vi "cleanWaypoints.vi"(10 "Waypoint Queue":refnum<queue>, 11 "Old Waypoints":refnum<class "Waypoint.lvclass">[](array[class])) -> (2 "Done?":bool, 3 "Old Waypoints (updated)":refnum<class "Waypoint.lvclass">[](array[class]))   [LabVIEW 2013]
doc: "When the next waypoints has been marked done, remove it from the queue and add it to the waypoint history array"
uses:
  Logic/Classes/Waypoint/Waypoint.lvclass
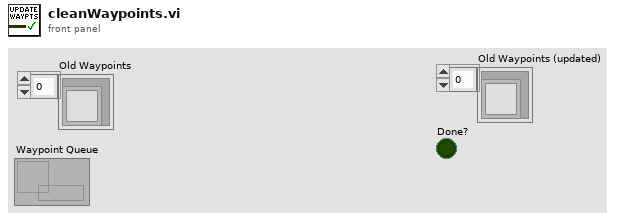
[diagram p1: front panel]
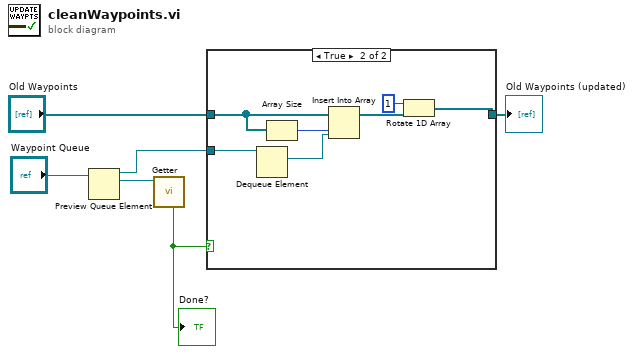
[diagram p0: block diagram]
diagram:
  n1 = Preview Queue Element(queue="Waypoint Queue") -> (queue out=w3:refnum<queue>, element=w5:refnum<class "Waypoint.lvclass">)  [unwired: 2 in, 2 out]
  n2 = call "Getter.vi"("Waypoint In"=w5) -> ("Done?"=w4:bool)  [unwired: 6 in, 4 out]
  "Done?" <- w4
  n3 = case shown="True" w4 {
    tunnel: w3 -> [_ w14]
    tunnel: "Old Waypoints" -> [w7 w12]
    tunnel: [w7 w8] -> w1
    frame False {
    }
    frame True {
      n4 = Dequeue Element(queue=w14) -> (element=w13:refnum<class "Waypoint.lvclass">)  [unwired: 2 in, 3 out]
      n5 = Array Size(array=w12) -> (size(s)=w11:i32)
      n6 = Insert Into Array(array=w12, index=w11, new element=w13) -> (w10:refnum<class "Waypoint.lvclass">[])
      n7 = Rotate 1D Array(1:w10, 2:1 ("n")) -> (0:w8:refnum<class "Waypoint.lvclass">[])
    }
  }
  "Old Waypoints (updated)" <- w1
